vi "PH_4_Pos_Selector.destructor.vi"(0 "i ref in":refnum<vi>, 5 "error in(no error)":errorcluster) -> (19 "error out":errorcluster)   [LabVIEW 2014, in "PH_4_Pos_Selector.lvlib"]
doc: "This is the destructor of a class.\n\nLicense Agreement for this software:\n\nCopyright (C)\nGesellschaft für Schwerionenforschung, GSI\nPlanckstr. 1\n64291 Darmstadt\nGermany\n\nContact: D.Beck@gsi.de \n\nThis program is free software; you can redistribute it and/or modify it under the terms of the \nGNU General Public License as published by the Free Software Foundation; either version 2 of \nthe license, or (at your option) any later version.\n\nThis program is distributed in the hope that it will be useful, but WITHOUT ANY WARRANTY; \nwithout even the implied warranty of MERCHANTABILITY or FITNESS FOR A PARTICULAR PURPOSE. See the GNU General License for more details (http://www.gnu.org).\n\nGesellschaft für Schwerionenforschung, GSI\nPlanckstr. 1, 64291 Darmstadt, Germany\nFor all questions and ideas contact: M.Richter@gsi.de, H.Brand@gsi.de or D.Beck@gsi.de.\nLast update: 16-JUN-2004"
uses:
  PH_4_Pos_Selector.lvlib
  PH_AxisGUI_6P/PH_AxisGUI_6P.lvlib
  lib.lib/DimLVEvent/LVDimInterface/LVDimInterface.lvlib
  PH_PSDBWriter/PH_PSDBWriter.lvlib
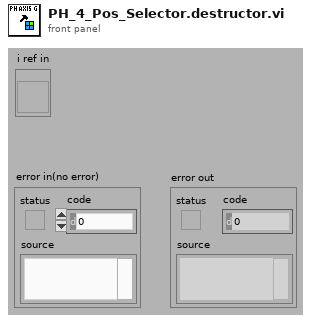
[diagram p1: front panel]
types:
  T1 = typedef "PH_4_Pos_Selector.lvlib/PH_4_Pos_Selector.i attribute.ctl" = cluster{"GUI Refs":cluster{"Position I":refnum<vi>, "Position II":refnum<vi>, "Position III":refnum<vi>, "Position IV":refnum<vi>, "rel. Mode?":refnum<vi>, "Define Selector":refnum<vi>}, "Current Position":T2, "Service ID Position":i32, "Position Array":T3[], "Description Array":string[], "relative Mode":bool, "Wanted Define Selector Position":string}
  T2 = typedef "PH_4_Pos_Selector.lvlib/PH_4_Pos_Selector.Position Selector.ctl" = u16
  T3 = typedef "PH_4_Pos_Selector.lvlib/PH_4_Pos_Selector.Position.ctl" = cluster{"Axis 1":dbl, "Axis 2":dbl}
  T4 = enum16{"SetAttribute", "GetAttribute", "CreateAttribute", "DestroyAttribute", "DestroyAllAtributes"}
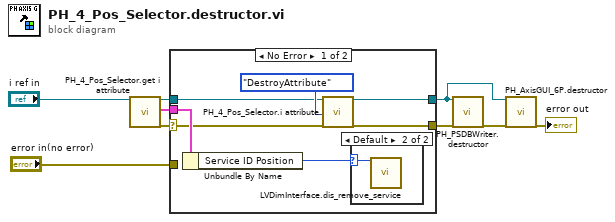
[diagram p0: block diagram]
diagram:
  n1 = call "PH_4_Pos_Selector.get i attribute.vi"("i ref in"="i ref in") -> ("i ref out"=w8:refnum<vi>, "i attribute"=w7:T1, "error out"=w3:errorcluster)  [unwired: 16 in]
  n2 = case shown="No Error" w3 {
    selector: w3 -> [w10 _]
    tunnel: w8 -> [w15 w19]
    tunnel: w7 -> [w14 _]
    tunnel: [w12 w18] -> w6
    tunnel: [w11 w19] -> w4
    tunnel: "error in(no error)" -> [_ w18]
    frame No Error {
      n3 = Unbundle By Name(w14) -> ("Service ID Position"=w13:i32)
      n4 = call "PH_4_Pos_Selector.i attribute.vi"("VI Refnum"=w15, "Action"=T4."DestroyAttribute", "error in (no error)"=w10) -> ("VI Refnum out"=w11:refnum<vi>, "error out"=w12:errorcluster)  [unwired: 14 in, 1 out]
      n5 = case shown="Default" w13 {
        selector: w13 -> [_ w17]
        frame -1 {
        }
        frame Default {
          n6 = call "LVDimInterface.dis_remove_service.vi"("my_serviceID"=w17) -> ()  [unwired: 18 in, 1 out]
        }
      }
    }
    frame Error {
    }
  }
  n7 = call "PH_PSDBWriter.destructor.vi"("i ref in"=w4, "error in(no error)"=w6) -> ("error out"=w5:errorcluster)  [unwired: 17 in]
  n8 = call "PH_AxisGUI_6P.destructor.vi"("i ref in"=w4, "error in(no error)"=w5) -> ("error out"=→"error out":errorcluster)  [unwired: 17 in]
